vi "temperature_logger.vi"() -> ()   [LabVIEW 2017]
panel:
  out "Temperature Log":string
  out "Thermometer":dbl(slide) scale=0.0..100.0
  out "x+1":i32
  out "time stamp":timestamp
  out "date/time string":string
  in  "stop":bool
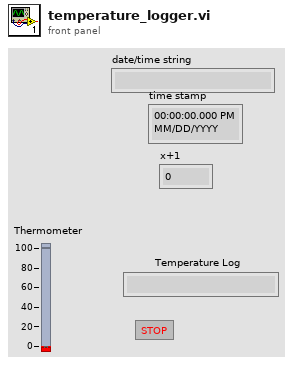
[diagram p1: front panel]
types:
  T1 = typedef "LVDateTimeRec.ctl" = cluster{"fractional second":dbl, "second":i32, "minute":i32, "hour":i32, "day of month":i32, "month":i32, "year":i32, "day of week":i32, "day of year":i32, "DST":i32}
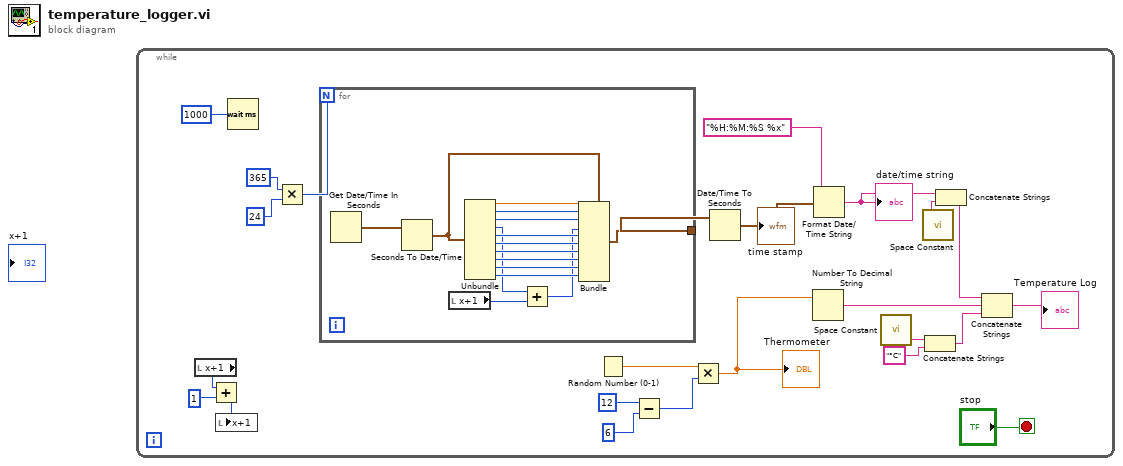
[diagram p0: block diagram]
diagram:
  n1 = while {
    stop <- "stop" stop-if-true
    n2 = local read "x+1"() -> (w16:i32)
    n3 = Add(x=w16, y=1) -> (x+y=w15:i32)
    n4 = local write "x+1"(w15) -> ()
    n5 = Wait (ms)(milliseconds to wait=u32 1000) -> ()  [unwired: 1 out]
    n6 = Multiply(x=365, y=24) -> (x*y=w22:i32)
    n7 = for {
      N: w22 -> [_]
      tunnel: [w30] -> w18
      n8 = Get Date/Time In Seconds() -> (seconds since 1Jan1904=w29:timestamp)
      n9 = Seconds To Date/Time(time stamp (now)=w29) -> (date time rec=w28:T1)  [unwired: 1 in]
      n10 = local read "x+1"() -> (w25:i32)
      n11 = Unbundle(w28) -> ("fractional second"=w39:dbl, "second"=w38:i32, "minute"=w37:i32, "hour"=w27:i32, "day of month"=w36:i32, "month"=w35:i32, "year"=w34:i32, "day of week"=w33:i32, "day of year"=w32:i32, "DST"=w31:i32)
      n12 = Add(x=w27, y=w25) -> (x+y=w26:i32)
      n13 = Bundle(cluster=w28, "fractional second"=w39, "second"=w38, "minute"=w37, "hour"=w26, "day of month"=w36, "month"=w35, "year"=w34, "day of week"=w33, "day of year"=w32, "DST"=w31) -> (w30:T1)
    }
    n14 = Random Number (0-1)() -> (number: 0 to 1=w5:dbl)
    n15 = Subtract(x=12, y=6) -> (x-y=w2:i32)
    n16 = Multiply(x=w5, y=w2) -> (x*y=w1:dbl)
    "Thermometer" <- w1
    n17 = Date/Time To Seconds(2:w18) -> (0:w19:timestamp)  [unwired: 1 in]
    "time stamp" <- w19
    n18 = Number To Decimal String(number=w1) -> (decimal integer string=w14:string)  [unwired: 1 in]
    n19 = Format Date/Time String(time format string (%c)="%H:%M:%S %x", seconds (now)=w19) -> (date/time string=w12:string)  [unwired: 1 in]
    "date/time string" <- w12
    n20 = call <vilib>:"Space Constant.vi"() -> ("String"=w8:string)
    n21 = call <vilib>:"Space Constant.vi"() -> ("String"=w13:string)
    n22 = Concatenate Strings(w8, "°C") -> (w6:string)
    n23 = Concatenate Strings(w12, w13) -> (w11:string)
    n24 = Concatenate Strings(w11, w14, w6) -> (→"Temperature Log":string)
  }
